vi "ConvTempTlog.vi"(4 "error in":errorcluster, 6 "NouvDonnées Y":dbl[](array[numeric]), 7 "TablesConv":u16[](array[numeric]) caption="No Courbe de conversion" max=60 step=1) -> (0 "error out":errorcluster, 2 "NouvDonnées Y Out":dbl[](array[numeric]))   [LabVIEW 2010]
doc: "Ce Vi prend un tableau de donnée et convertit chaque donées selon la fonction spécifié par l'indicateur du même index dans la table de conversion."
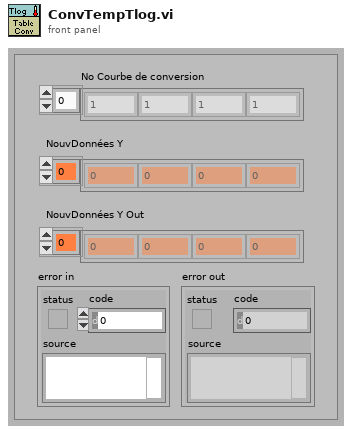
[diagram p1: front panel]
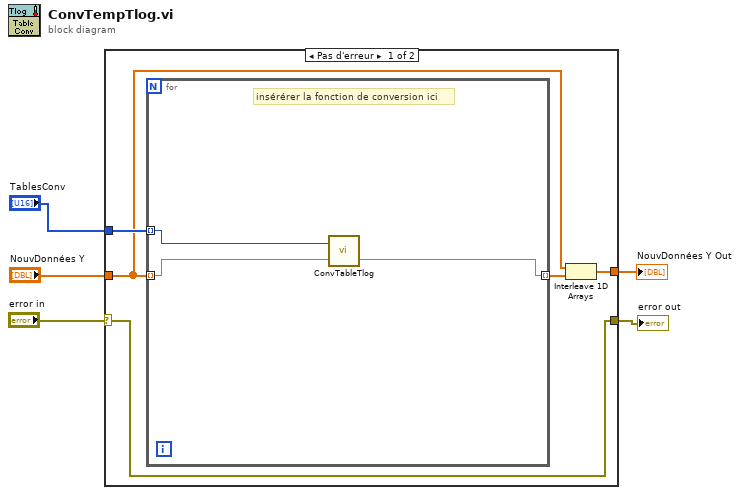
[diagram p0: block diagram]
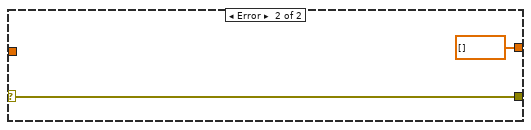
[diagram p2: hidden frame]
diagram:
  n1 = case shown="Pas d'erreur" "error in" {
    selector: "error in" -> [w6 w15]
    tunnel: "TablesConv" -> [w10 _]
    tunnel: "NouvDonnées Y" -> [w8 _]
    tunnel: [w7 dbl[] []] -> w3
    tunnel: [w6 w15] -> w1
    frame No Error {
      n2 = for {
        tunnel: w8 -> [w12] mode=indexing
        tunnel: w10 -> [w13] mode=indexing
        tunnel: [w11] -> w9 mode=indexing
        # "insérérer la fonction de conversion ici"
        n3 = call <userlib>:"ConvTableTlog.vi"("Mesure"=w12, "Courbe conversion"=w13) -> ("Température"=w11:dbl)  [unwired: 1 out]
      }
      n4 = Interleave 1D Arrays(w8, w9) -> (w7:dbl[])
    }
    frame Error {
    }
  }
  "NouvDonnées Y Out" <- w3
  "error out" <- w1
